vi "Modbus ASCII String to Byte Array.vi"(11 "string":string) -> (3 "byte array":u8[](array[numeric]))   [LabVIEW 2020, in "Library Instrument & Equipement.lvlib" / "Library Relay_Board.lvlib" / "Modbus.lvclass"]
doc: "Converts Modbus ASCII <B>string</B> to <B>byte array</B>."
uses:
  Modbus.lvclass
  Modbus.lvclass/Modbus.ctl
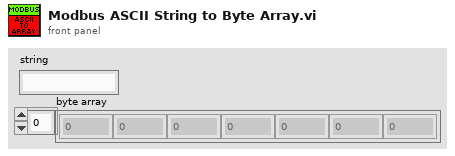
[diagram p1: front panel]
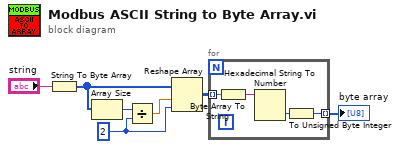
[diagram p0: block diagram]
diagram:
  w6 = 2 ("y")
  n1 = String To Byte Array(string="string") -> (unsigned byte array=w3:u8[])
  n2 = Array Size(array=w3) -> (size(s)=w4:i32)
  n3 = Divide(x=w4, y=w6) -> (x/y=w5:dbl)
  n4 = Reshape Array(w3, w5, w6) -> (w7:u8[][])
  n5 = for {
    tunnel: w7 -> [w11] mode=indexing
    tunnel: [w8] -> w2 mode=indexing
    n6 = Byte Array To String(unsigned byte array=w11) -> (string=w10:string)
    n7 = Hexadecimal String To Number(string=w10) -> (number=w9:u32)  [unwired: 2 in, 1 out]
    n8 = To Unsigned Byte Integer(number=w9) -> (unsigned 8bit integer=w8:u8)
  }
  "byte array" <- w2
